vi "ConfigureAcquisition.vi"(8 "error in (no error)":errorcluster, 11 "Infiniium in":refnum<class "Infiniium.lvclass">) -> (0 "error out":errorcluster, 3 "Infiniium out":refnum<class "Infiniium.lvclass">)   [LabVIEW 2018]
uses:
  <instrlib>/Agilent 90000 Series/Agilent 90000 Series.lvlib
  Infiniium.lvclass
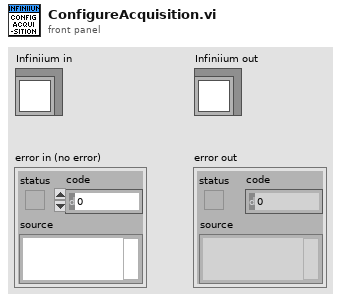
[diagram p1: front panel]
types:
  T1 = typedef "ScopePlugins.lvlib/Acquisition.ctl" = cluster{"StartTime":dbl, "Type":enum16{"Normal", "PeakDetect", "HighRes", "Envelope", "Average"}, "NumPointsMin":i32, "RecordLength":i32, "SampleRate":dbl, "TimePerRecord":dbl, "SamplingMode ":enum16{"Real Time", "Equivalent Time", "Segment", "Real Time Peak Detect", "Real Time High Resolution", "Peak Detect Segment", "High Resolution Segment"}, "Interpolation":enum16{"No Interpolation", "sin(x)/x", "linear", "1 Point sin(x)/x", "2 Point sin(x)/x", "4 Point sin(x)/x", "8 Point sin(x)/x", "16 Point sin(x)/x"}, "NumAverages":i32, "Resolution":enum16{"Auto", "Bits 9", "Bits 10", "Bits 11", "Bits 12"}, "EnableAveraging":bool, "Continuous":bool}
  T2 = enum16{"Normal", "PeakDetect", "HighRes", "Envelope", "Average"}
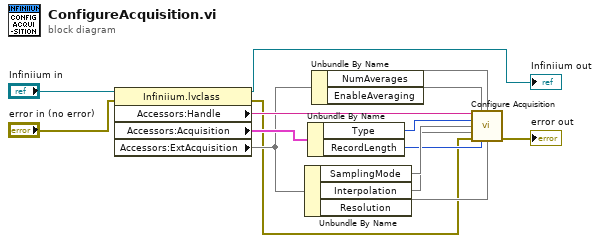
[diagram p0: block diagram]
diagram:
  n1 = property class="Infiniium.lvclass"(reference="Infiniium in", error in="error in (no error)") -> (reference out=→"Infiniium out":refnum<class "Infiniium.lvclass">, error out=w3:errorcluster, "Accessors:Handle"=w13:string, "Accessors:Acquisition"=w12:T1, "Accessors:ExtAcquisition"=w7)
  n2 = Unbundle By Name(w7) -> ("SamplingMode"=w10, "Interpolation"=w9, "Resolution"=w4)
  n3 = Unbundle By Name(w12) -> ("Type"=w11:T2, "RecordLength"=w8:i32)
  n4 = Unbundle By Name(w7) -> ("NumAverages"=w6, "EnableAveraging"=w5)
  n5 = call <instrlib>:"Configure Acquisition.vi"("VISA resource name"=w13, "Enable Analog Averaging (Disable)"=w5, "Number Of Averages (8)"=w6, "Acquisition Type (0: Normal)"=w11, "Sampling Mode  (0: Real Time)"=w10, "Interpolation (0:No Interpolation)"=w9, "error in (no error)"=w3, "Segment Count (256)"=w8, "Resolution (0:Auto)"=w4) -> ("error out"=→"error out":errorcluster)  [unwired: 5 in, 1 out]
